vi "set_LM_states.vi"(8 "error in (no error)":errorcluster caption="错误输入（无错误）", 10 "LM states":cluster{"state -":bool, "state +":bool}[](array[cluster]), 11 "MotorSystem 输入":refnum<class "MotorSystem.lvclass">) -> (0 "error out":errorcluster caption="错误输出", 3 "MotorSystem 输出":refnum<class "MotorSystem.lvclass">)   [LabVIEW 2014, in "MotorSystem.lvclass"]
uses:
  MotorSystem.lvclass
  MotorSystem.lvclass/MotorSystem.ctl
  OneMotion/OneMotion.lvclass/OneMotion.ctl
  LimitSwitch/LimitSwitch.lvclass/LimitSwitch.ctl
  OneMotion/OneMotion.lvclass
  LimitSwitch/LimitSwitch.lvclass
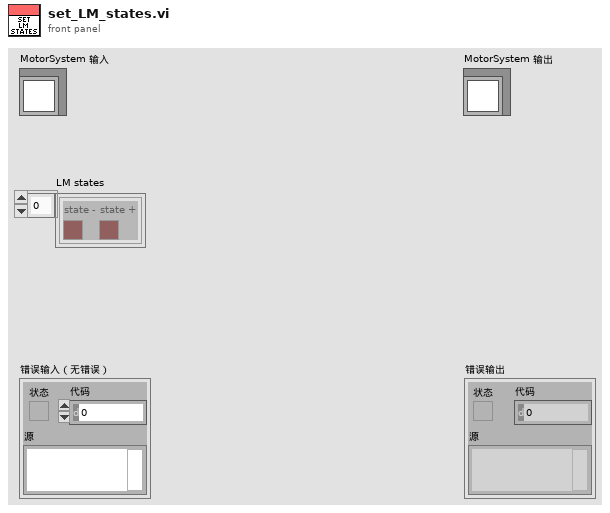
[diagram p1: front panel]
types:
  T1 = typedef "MotorSystem.lvclass/MotionCluster.ctl" = cluster{"OneMotion.lvclass":refnum<class "OneMotion.lvclass">, "connected?":bool, "default enabled?":bool, "enabled?":bool}
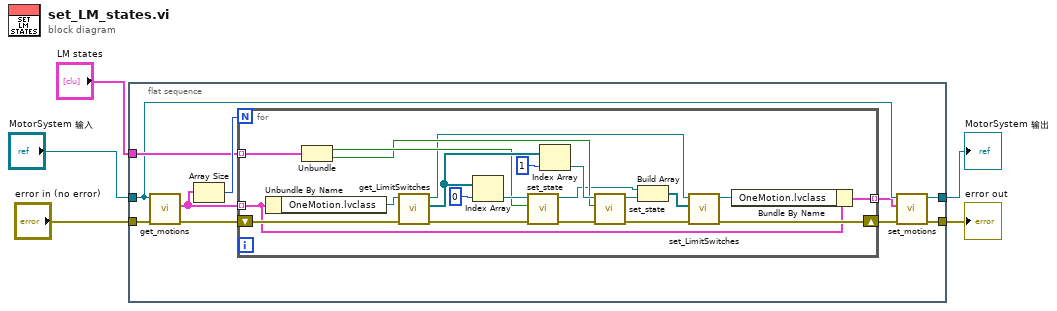
[diagram p0: block diagram]
diagram:
  n1 = flat-sequence {
    tunnel: [w6] -> w5
    tunnel: [w9] -> w3
    tunnel: "MotorSystem 输入" -> [w10]
    tunnel: "error in (no error)" -> [w13]
    tunnel: "LM states" -> [w11]
    frame #0 {
      n2 = call "get_motions.vi"("error in (no error)"=w13, "MotorSystem输入"=w10) -> ("error out"=w12:errorcluster, "motions"=w14:T1[])  [unwired: 7 in, 1 out]
      n3 = Array Size(array=w14) -> (size(s)=w15:i32)
      n4 = for {
        N: w15 -> [_]
        tunnel: w14 -> [w18] mode=indexing
        shift-right: [w19] -> w7
        shift-left: w12 -> [w32]
        tunnel: w11 -> [w31] mode=indexing
        tunnel: [w16] -> w8 mode=indexing
        n5 = Unbundle By Name(w18) -> ("OneMotion.lvclass"=w36:refnum<class "OneMotion.lvclass">)
        n6 = Unbundle(w31) -> ("state -"=w26:bool, "state +"=w25:bool)
        n7 = call "get_LimitSwitches.vi"("error in (no error)"=w32, "OneMotion输入"=w36) -> ("error out"=w28:errorcluster, "LimitSwitches"=w33:refnum<class "LimitSwitch.lvclass">[], "OneMotion输出"=w22:refnum<class "OneMotion.lvclass">)  [unwired: 7 in]
        n8 = Index Array(array=w33, index=0 ("索引")) -> (element=w30:refnum<class "LimitSwitch.lvclass">)
        n9 = call "set_state.vi"("error in (no error)"=w28, "state"=w26, "LimitSwitch输入"=w30) -> ("error out"=w27:errorcluster, "LimitSwitch输出"=w24:refnum<class "LimitSwitch.lvclass">)  [unwired: 7 in]
        n10 = Index Array(array=w33, index=1 ("索引")) -> (element=w29:refnum<class "LimitSwitch.lvclass">)
        n11 = call "set_state.vi"("error in (no error)"=w27, "state"=w25, "LimitSwitch输入"=w29) -> ("error out"=w20:errorcluster, "LimitSwitch输出"=w23:refnum<class "LimitSwitch.lvclass">)  [unwired: 7 in]
        n12 = Build Array(w24, w23) -> (w21:refnum<class "LimitSwitch.lvclass">[])
        n13 = call "set_LimitSwitches.vi"("error in (no error)"=w20, "LimitSwitches"=w21, "OneMotion输入"=w22) -> ("error out"=w19:errorcluster, "OneMotion输出"=w17:refnum<class "OneMotion.lvclass">)  [unwired: 7 in]
        n14 = Bundle By Name(cluster=w18, "OneMotion.lvclass"=w17) -> (w16:T1)
      }
      n15 = call "set_motions.vi"("error in (no error)"=w7, "motions"=w8, "MotorSystem输入"=w10) -> ("error out"=w6:errorcluster, "MotorSystem输出"=w9:refnum<class "MotorSystem.lvclass">)  [unwired: 7 in]
    }
  }
  "error out" <- w5
  "MotorSystem 输出" <- w3
